vi "fetch frame gige DB1605 无点云.vi"() -> ()   [LabVIEW 2015]
uses:
  <userlib>/Mv3dRgbd/Mv3dRgbd.lvlib
  <userlib>/Mv3dRgbdEx/Mv3dRgbdEx.lvlib
panel:
  in  "设备索引":i32=5
  out "pDeviceCount out 4":u32
  out "get list return 3":i32
  out "MV3D_RGBD_GigEDEVICE_INFO out 3":T1(array[cluster])
  out "pstGigeDeviceInfo out 3":T2
  out "open gige function 2":i32
  out "start handle out":u32
  out "start function 2":i32
  in  "?":enum32{"RGBD", "点云"}(tab)
  out "二维图片":picture
  out "Depth":i16[][](graph)
  out "fetchframe function":i32
  in  "?":bool
  out "close handle out":u32
  out "close function":i32
  out "stop handle out":u32
  out "init function":i32
  out "release function":i32
  out "stop function":i32
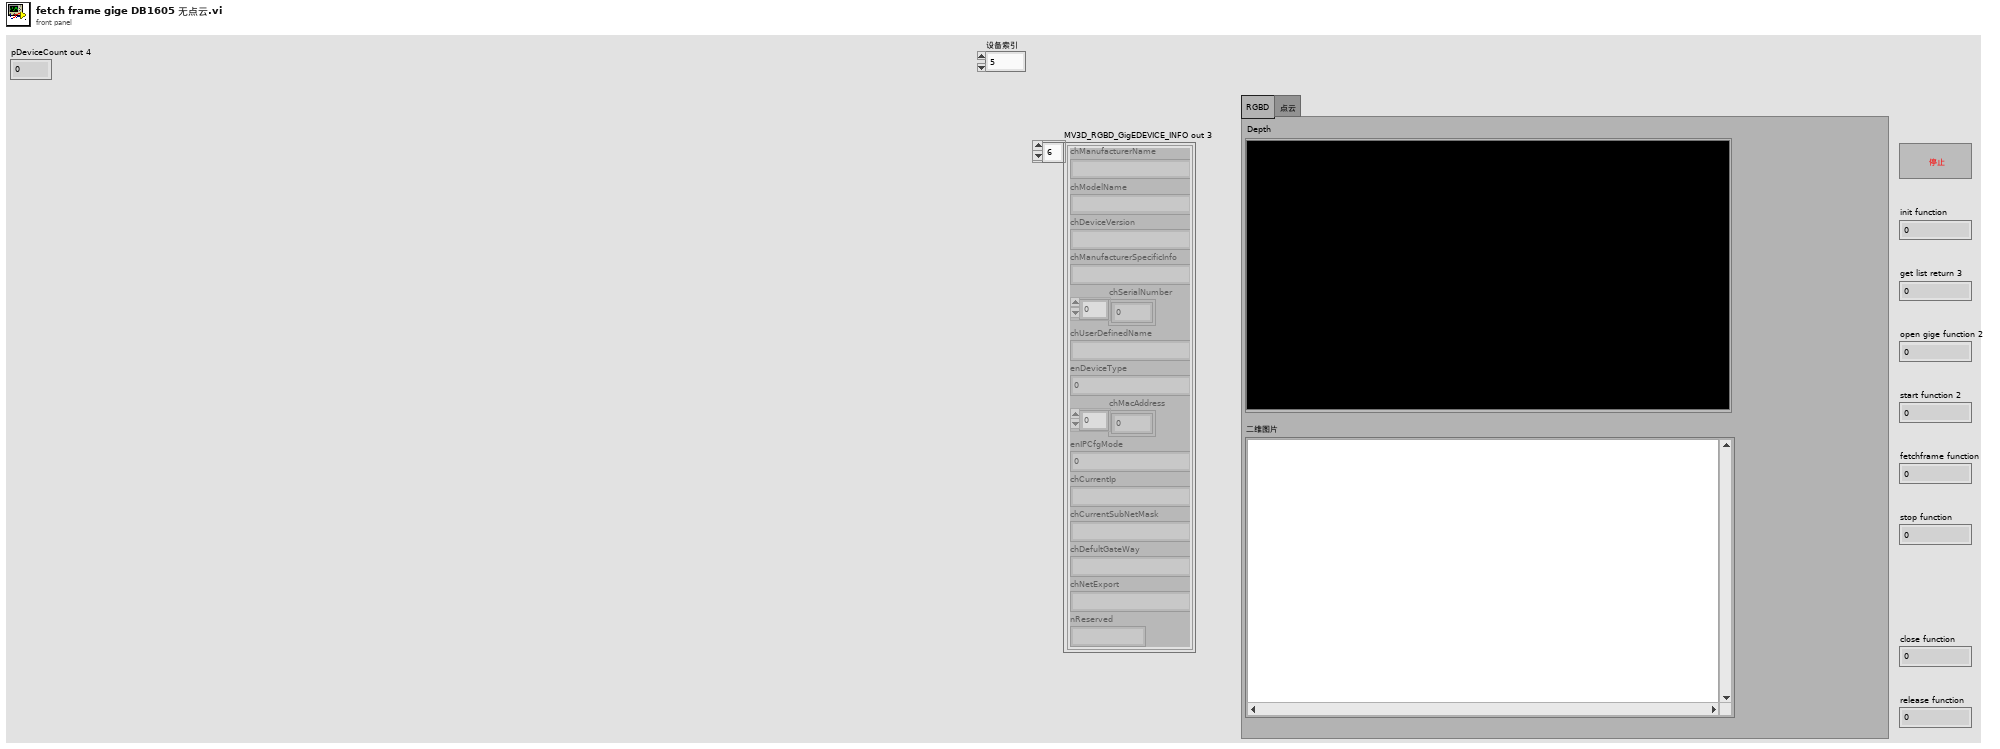
[diagram p1: front panel]
types:
  T1 = cluster{"chManufacturerName":string, "chModelName":string, "chDeviceVersion":string, "chManufacturerSpecificInfo":string, "chSerialNumber":u8[], "chUserDefinedName":string, "enDeviceType":i32, "chMacAddress":u8[], "enIPCfgMode":i32, "chCurrentIp":string, "chCurrentSubNetMask":string, "chDefultGateWay":string, "chNetExport":string, "nReserved":string}[]
  T2 = cluster{"chManufacturerName[0]":i8, "chManufacturerName[1]":i8, "chManufacturerName[2]":i8, "chManufacturerName[3]":i8, "chManufacturerName[4]":i8, "chManufacturerName[5]":i8, "chManufacturerName[6]":i8, "chManufacturerName[7]":i8, "chManufacturerName[8]":i8, "chManufacturerName[9]":i8, "chManufacturerName[10]":i8, "chManufacturerName[11]":i8, "chManufacturerName[12]":i8, "chManufacturerName[13]":i8, "chManufacturerName[14]":i8, "chManufacturerName[15]":i8, "chManufacturerName[16]":i8, "chManufacturerName[17]":i8, "chManufacturerName[18]":i8, "chManufacturerName[19]":i8, "chManufacturerName[20]":i8, "chManufacturerName[21]":i8, "chManufacturerName[22]":i8, "chManufacturerName[23]":i8, "chManufacturerName[24]":i8, "chManufacturerName[25]":i8, "chManufacturerName[26]":i8, "chManufacturerName[27]":i8, "chManufacturerName[28]":i8, "chManufacturerName[29]":i8, "chManufacturerName[30]":i8, "chManufacturerName[31]":i8, "chModelName[0]":i8, "chModelName[1]":i8, "chModelName[2]":i8, "chModelName[3]":i8, "chModelName[4]":i8, "chModelName[5]":i8, "chModelName[6]":i8, "chModelName[7]":i8, "chModelName[8]":i8, "chModelName[9]":i8, "chModelName[10]":i8, "chModelName[11]":i8, "chModelName[12]":i8, "chModelName[13]":i8, "chModelName[14]":i8, "chModelName[15]":i8, "chModelName[16]":i8, "chModelName[17]":i8, "chModelName[18]":i8, "chModelName[19]":i8, "chModelName[20]":i8, "chModelName[21]":i8, "chModelName[22]":i8, "chModelName[23]":i8, "chModelName[24]":i8, "chModelName[25]":i8, "chModelName[26]":i8, "chModelName[27]":i8, "chModelName[28]":i8, "chModelName[29]":i8, "chModelName[30]":i8, "chModelName[31]":i8, "chDeviceVersion[0]":i8, "chDeviceVersion[1]":i8, "chDeviceVersion[2]":i8, "chDeviceVersion[3]":i8, "chDeviceVersion[4]":i8, "chDeviceVersion[5]":i8, "chDeviceVersion[6]":i8, "chDeviceVersion[7]":i8, "chDeviceVersion[8]":i8, "chDeviceVersion[9]":i8, "chDeviceVersion[10]":i8, "chDeviceVersion[11]":i8, "chDeviceVersion[12]":i8, "chDeviceVersion[13]":i8, "chDeviceVersion[14]":i8, "chDeviceVersion[15]":i8, "chDeviceVersion[16]":i8, "chDeviceVersion[17]":i8, "chDeviceVersion[18]":i8, "chDeviceVersion[19]":i8, "chDeviceVersion[20]":i8, "chDeviceVersion[21]":i8, "chDeviceVersion[22]":i8, "chDeviceVersion[23]":i8, "chDeviceVersion[24]":i8, "chDeviceVersion[25]":i8, "chDeviceVersion[26]":i8, "chDeviceVersion[27]":i8, "chDeviceVersion[28]":i8, "chDeviceVersion[29]":i8, "chDeviceVersion[30]":i8, "chDeviceVersion[31]":i8, "chManufacturerSpecificInfo[0]":i8, "chManufacturerSpecificInfo[1]":i8, "chManufacturerSpecificInfo[2]":i8, "chManufacturerSpecificInfo[3]":i8, "chManufacturerSpecificInfo[4]":i8, "chManufacturerSpecificInfo[5]":i8, "chManufacturerSpecificInfo[6]":i8, "chManufacturerSpecificInfo[7]":i8, "chManufacturerSpecificInfo[8]":i8, "chManufacturerSpecificInfo[9]":i8, "chManufacturerSpecificInfo[10]":i8, "chManufacturerSpecificInfo[11]":i8, "chManufacturerSpecificInfo[12]":i8, "chManufacturerSpecificInfo[13]":i8, "chManufacturerSpecificInfo[14]":i8, "chManufacturerSpecificInfo[15]":i8, "chManufacturerSpecificInfo[16]":i8, "chManufacturerSpecificInfo[17]":i8, "chManufacturerSpecificInfo[18]":i8, "chManufacturerSpecificInfo[19]":i8, "chManufacturerSpecificInfo[20]":i8, "chManufacturerSpecificInfo[21]":i8, "chManufacturerSpecificInfo[22]":i8, "chManufacturerSpecificInfo[23]":i8, "chManufacturerSpecificInfo[24]":i8, "chManufacturerSpecificInfo[25]":i8, "chManufacturerSpecificInfo[26]":i8, "chManufacturerSpecificInfo[27]":i8, "chManufacturerSpecificInfo[28]":i8, "chManufacturerSpecificInfo[29]":i8, "chManufacturerSpecificInfo[30]":i8, "chManufacturerSpecificInfo[31]":i8, "chManufacturerSpecificInfo[32]":i8, "chManufacturerSpecificInfo[33]":i8, "chManufacturerSpecificInfo[34]":i8, "chManufacturerSpecificInfo[35]":i8, "chManufacturerSpecificInfo[36]":i8, "chManufacturerSpecificInfo[37]":i8, "chManufacturerSpecificInfo[38]":i8, "chManufacturerSpecificInfo[39]":i8, "chManufacturerSpecificInfo[40]":i8, "chManufacturerSpecificInfo[41]":i8, "chManufacturerSpecificInfo[42]":i8, "chManufacturerSpecificInfo[43]":i8, "chManufacturerSpecificInfo[44]":i8, "chManufacturerSpecificInfo[45]":i8, "chManufacturerSpecificInfo[46]":i8, "chManufacturerSpecificInfo[47]":i8, "chSerialNumber[0]":i8, "chSerialNumber[1]":i8, "chSerialNumber[2]":i8, "chSerialNumber[3]":i8, "chSerialNumber[4]":i8, "chSerialNumber[5]":i8, "chSerialNumber[6]":i8, "chSerialNumber[7]":i8, "chSerialNumber[8]":i8, "chSerialNumber[9]":i8, "chSerialNumber[10]":i8, "chSerialNumber[11]":i8, "chSerialNumber[12]":i8, "chSerialNumber[13]":i8, "chSerialNumber[14]":i8, "chSerialNumber[15]":i8, "chUserDefinedName[0]":i8, "chUserDefinedName[1]":i8, "chUserDefinedName[2]":i8, "chUserDefinedName[3]":i8, "chUserDefinedName[4]":i8, "chUserDefinedName[5]":i8, "chUserDefinedName[6]":i8, "chUserDefinedName[7]":i8, "chUserDefinedName[8]":i8, "chUserDefinedName[9]":i8, "chUserDefinedName[10]":i8, "chUserDefinedName[11]":i8, "chUserDefinedName[12]":i8, "chUserDefinedName[13]":i8, "chUserDefinedName[14]":i8, "chUserDefinedName[15]":i8, "enDeviceType":i32, "chMacAddress[0]":u8, "chMacAddress[1]":u8, "chMacAddress[2]":u8, "chMacAddress[3]":u8, "chMacAddress[4]":u8, "chMacAddress[5]":u8, "chMacAddress[6]":u8, "chMacAddress[7]":u8, "enIPCfgMode":i32, "chCurrentIp[0]":i8, "chCurrentIp[1]":i8, "chCurrentIp[2]":i8, "chCurrentIp[3]":i8, "chCurrentIp[4]":i8, "chCurrentIp[5]":i8, "chCurrentIp[6]":i8, "chCurrentIp[7]":i8, "chCurrentIp[8]":i8, "chCurrentIp[9]":i8, "chCurrentIp[10]":i8, "chCurrentIp[11]":i8, "chCurrentIp[12]":i8, "chCurrentIp[13]":i8, "chCurrentIp[14]":i8, "chCurrentIp[15]":i8, "chCurrentSubNetMask[0]":i8, "chCurrentSubNetMask[1]":i8, "chCurrentSubNetMask[2]":i8, "chCurrentSubNetMask[3]":i8, "chCurrentSubNetMask[4]":i8, "chCurrentSubNetMask[5]":i8, "chCurrentSubNetMask[6]":i8, "chCurrentSubNetMask[7]":i8, "chCurrentSubNetMask[8]":i8, "chCurrentSubNetMask[9]":i8, "chCurrentSubNetMask[10]":i8, "chCurrentSubNetMask[11]":i8, "chCurrentSubNetMask[12]":i8, "chCurrentSubNetMask[13]":i8, "chCurrentSubNetMask[14]":i8, "chCurrentSubNetMask[15]":i8, "chDefultGateWay[0]":i8, "chDefultGateWay[1]":i8, "chDefultGateWay[2]":i8, "chDefultGateWay[3]":i8, "chDefultGateWay[4]":i8, "chDefultGateWay[5]":i8, "chDefultGateWay[6]":i8, "chDefultGateWay[7]":i8, "chDefultGateWay[8]":i8, "chDefultGateWay[9]":i8, "chDefultGateWay[10]":i8, "chDefultGateWay[11]":i8, "chDefultGateWay[12]":i8, "chDefultGateWay[13]":i8, "chDefultGateWay[14]":i8, "chDefultGateWay[15]":i8, "chNetExport[0]":i8, "chNetExport[1]":i8, "chNetExport[2]":i8, "chNetExport[3]":i8, "chNetExport[4]":i8, "chNetExport[5]":i8, "chNetExport[6]":i8, "chNetExport[7]":i8, "chNetExport[8]":i8, "chNetExport[9]":i8, "chNetExport[10]":i8, "chNetExport[11]":i8, "chNetExport[12]":i8, "chNetExport[13]":i8, "chNetExport[14]":i8, "chNetExport[15]":i8, "nReserved[0]":u8, "nReserved[1]":u8, "nReserved[2]":u8, "nReserved[3]":u8, "nReserved[4]":u8, "nReserved[5]":u8, "nReserved[6]":u8, "nReserved[7]":u8, "nReserved[8]":u8, "nReserved[9]":u8, "nReserved[10]":u8, "nReserved[11]":u8, "nReserved[12]":u8, "nReserved[13]":u8, "nReserved[14]":u8, "nReserved[15]":u8}
  T3 = cluster{"chManufacturerName[0]":i8, "chManufacturerName[1]":i8, "chManufacturerName[2]":i8, "chManufacturerName[3]":i8, "chManufacturerName[4]":i8, "chManufacturerName[5]":i8, "chManufacturerName[6]":i8, "chManufacturerName[7]":i8, "chManufacturerName[8]":i8, "chManufacturerName[9]":i8, "chManufacturerName[10]":i8, "chManufacturerName[11]":i8, "chManufacturerName[12]":i8, "chManufacturerName[13]":i8, "chManufacturerName[14]":i8, "chManufacturerName[15]":i8, "chManufacturerName[16]":i8, "chManufacturerName[17]":i8, "chManufacturerName[18]":i8, "chManufacturerName[19]":i8, "chManufacturerName[20]":i8, "chManufacturerName[21]":i8, "chManufacturerName[22]":i8, "chManufacturerName[23]":i8, "chManufacturerName[24]":i8, "chManufacturerName[25]":i8, "chManufacturerName[26]":i8, "chManufacturerName[27]":i8, "chManufacturerName[28]":i8, "chManufacturerName[29]":i8, "chManufacturerName[30]":i8, "chManufacturerName[31]":i8, "chModelName[0]":i8, "chModelName[1]":i8, "chModelName[2]":i8, "chModelName[3]":i8, "chModelName[4]":i8, "chModelName[5]":i8, "chModelName[6]":i8, "chModelName[7]":i8, "chModelName[8]":i8, "chModelName[9]":i8, "chModelName[10]":i8, "chModelName[11]":i8, "chModelName[12]":i8, "chModelName[13]":i8, "chModelName[14]":i8, "chModelName[15]":i8, "chModelName[16]":i8, "chModelName[17]":i8, "chModelName[18]":i8, "chModelName[19]":i8, "chModelName[20]":i8, "chModelName[21]":i8, "chModelName[22]":i8, "chModelName[23]":i8, "chModelName[24]":i8, "chModelName[25]":i8, "chModelName[26]":i8, "chModelName[27]":i8, "chModelName[28]":i8, "chModelName[29]":i8, "chModelName[30]":i8, "chModelName[31]":i8, "chDeviceVersion[0]":i8, "chDeviceVersion[1]":i8, "chDeviceVersion[2]":i8, "chDeviceVersion[3]":i8, "chDeviceVersion[4]":i8, "chDeviceVersion[5]":i8, "chDeviceVersion[6]":i8, "chDeviceVersion[7]":i8, "chDeviceVersion[8]":i8, "chDeviceVersion[9]":i8, "chDeviceVersion[10]":i8, "chDeviceVersion[11]":i8, "chDeviceVersion[12]":i8, "chDeviceVersion[13]":i8, "chDeviceVersion[14]":i8, "chDeviceVersion[15]":i8, "chDeviceVersion[16]":i8, "chDeviceVersion[17]":i8, "chDeviceVersion[18]":i8, "chDeviceVersion[19]":i8, "chDeviceVersion[20]":i8, "chDeviceVersion[21]":i8, "chDeviceVersion[22]":i8, "chDeviceVersion[23]":i8, "chDeviceVersion[24]":i8, "chDeviceVersion[25]":i8, "chDeviceVersion[26]":i8, "chDeviceVersion[27]":i8, "chDeviceVersion[28]":i8, "chDeviceVersion[29]":i8, "chDeviceVersion[30]":i8, "chDeviceVersion[31]":i8, "chManufacturerSpecificInfo[0]":i8, "chManufacturerSpecificInfo[1]":i8, "chManufacturerSpecificInfo[2]":i8, "chManufacturerSpecificInfo[3]":i8, "chManufacturerSpecificInfo[4]":i8, "chManufacturerSpecificInfo[5]":i8, "chManufacturerSpecificInfo[6]":i8, "chManufacturerSpecificInfo[7]":i8, "chManufacturerSpecificInfo[8]":i8, "chManufacturerSpecificInfo[9]":i8, "chManufacturerSpecificInfo[10]":i8, "chManufacturerSpecificInfo[11]":i8, "chManufacturerSpecificInfo[12]":i8, "chManufacturerSpecificInfo[13]":i8, "chManufacturerSpecificInfo[14]":i8, "chManufacturerSpecificInfo[15]":i8, "chManufacturerSpecificInfo[16]":i8, "chManufacturerSpecificInfo[17]":i8, "chManufacturerSpecificInfo[18]":i8, "chManufacturerSpecificInfo[19]":i8, "chManufacturerSpecificInfo[20]":i8, "chManufacturerSpecificInfo[21]":i8, "chManufacturerSpecificInfo[22]":i8, "chManufacturerSpecificInfo[23]":i8, "chManufacturerSpecificInfo[24]":i8, "chManufacturerSpecificInfo[25]":i8, "chManufacturerSpecificInfo[26]":i8, "chManufacturerSpecificInfo[27]":i8, "chManufacturerSpecificInfo[28]":i8, "chManufacturerSpecificInfo[29]":i8, "chManufacturerSpecificInfo[30]":i8, "chManufacturerSpecificInfo[31]":i8, "chManufacturerSpecificInfo[32]":i8, "chManufacturerSpecificInfo[33]":i8, "chManufacturerSpecificInfo[34]":i8, "chManufacturerSpecificInfo[35]":i8, "chManufacturerSpecificInfo[36]":i8, "chManufacturerSpecificInfo[37]":i8, "chManufacturerSpecificInfo[38]":i8, "chManufacturerSpecificInfo[39]":i8, "chManufacturerSpecificInfo[40]":i8, "chManufacturerSpecificInfo[41]":i8, "chManufacturerSpecificInfo[42]":i8, "chManufacturerSpecificInfo[43]":i8, "chManufacturerSpecificInfo[44]":i8, "chManufacturerSpecificInfo[45]":i8, "chManufacturerSpecificInfo[46]":i8, "chManufacturerSpecificInfo[47]":i8, "chSerialNumber[0]":i8, "chSerialNumber[1]":i8, "chSerialNumber[2]":i8, "chSerialNumber[3]":i8, "chSerialNumber[4]":i8, "chSerialNumber[5]":i8, "chSerialNumber[6]":i8, "chSerialNumber[7]":i8, "chSerialNumber[8]":i8, "chSerialNumber[9]":i8, "chSerialNumber[10]":i8, "chSerialNumber[11]":i8, "chSerialNumber[12]":i8, "chSerialNumber[13]":i8, "chSerialNumber[14]":i8, "chSerialNumber[15]":i8, "chUserDefinedName[0]":i8, "chUserDefinedName[1]":i8, "chUserDefinedName[2]":i8, "chUserDefinedName[3]":i8, "chUserDefinedName[4]":i8, "chUserDefinedName[5]":i8, "chUserDefinedName[6]":i8, "chUserDefinedName[7]":i8, "chUserDefinedName[8]":i8, "chUserDefinedName[9]":i8, "chUserDefinedName[10]":i8, "chUserDefinedName[11]":i8, "chUserDefinedName[12]":i8, "chUserDefinedName[13]":i8, "chUserDefinedName[14]":i8, "chUserDefinedName[15]":i8, "enDeviceType":i32, "chMacAddress[0]":u8, "chMacAddress[1]":u8, "chMacAddress[2]":u8, "chMacAddress[3]":u8, "chMacAddress[4]":u8, "chMacAddress[5]":u8, "chMacAddress[6]":u8, "chMacAddress[7]":u8, "enIPCfgMode":i32, "chCurrentIp[0]":i8, "chCurrentIp[1]":i8, "chCurrentIp[2]":i8, "chCurrentIp[3]":i8, "chCurrentIp[4]":i8, "chCurrentIp[5]":i8, "chCurrentIp[6]":i8, "chCurrentIp[7]":i8, "chCurrentIp[8]":i8, "chCurrentIp[9]":i8, "chCurrentIp[10]":i8, "chCurrentIp[11]":i8, "chCurrentIp[12]":i8, "chCurrentIp[13]":i8, "chCurrentIp[14]":i8, "chCurrentIp[15]":i8, "chCurrentSubNetMask[0]":i8, "chCurrentSubNetMask[1]":i8, "chCurrentSubNetMask[2]":i8, "chCurrentSubNetMask[3]":i8, "chCurrentSubNetMask[4]":i8, "chCurrentSubNetMask[5]":i8, "chCurrentSubNetMask[6]":i8, "chCurrentSubNetMask[7]":i8, "chCurrentSubNetMask[8]":i8, "chCurrentSubNetMask[9]":i8, "chCurrentSubNetMask[10]":i8, "chCurrentSubNetMask[11]":i8, "chCurrentSubNetMask[12]":i8, "chCurrentSubNetMask[13]":i8, "chCurrentSubNetMask[14]":i8, "chCurrentSubNetMask[15]":i8, "chDefultGateWay[0]":i8, "chDefultGateWay[1]":i8, "chDefultGateWay[2]":i8, "chDefultGateWay[3]":i8, "chDefultGateWay[4]":i8, "chDefultGateWay[5]":i8, "chDefultGateWay[6]":i8, "chDefultGateWay[7]":i8, "chDefultGateWay[8]":i8, "chDefultGateWay[9]":i8, "chDefultGateWay[10]":i8, "chDefultGateWay[11]":i8, "chDefultGateWay[12]":i8, "chDefultGateWay[13]":i8, "chDefultGateWay[14]":i8, "chDefultGateWay[15]":i8, "chNetExport[0]":i8, "chNetExport[1]":i8, "chNetExport[2]":i8, "chNetExport[3]":i8, "chNetExport[4]":i8, "chNetExport[5]":i8, "chNetExport[6]":i8, "chNetExport[7]":i8, "chNetExport[8]":i8, "chNetExport[9]":i8, "chNetExport[10]":i8, "chNetExport[11]":i8, "chNetExport[12]":i8, "chNetExport[13]":i8, "chNetExport[14]":i8, "chNetExport[15]":i8, "nReserved[0]":u8, "nReserved[1]":u8, "nReserved[2]":u8, "nReserved[3]":u8, "nReserved[4]":u8, "nReserved[5]":u8, "nReserved[6]":u8, "nReserved[7]":u8, "nReserved[8]":u8, "nReserved[9]":u8, "nReserved[10]":u8, "nReserved[11]":u8, "nReserved[12]":u8, "nReserved[13]":u8, "nReserved[14]":u8, "nReserved[15]":u8}[]
  T4 = cluster{"nImageCount":u64, "MV3D_RGBD_IMAGE_DATA[0]":cluster{"enImageType":i32, "nWidth":u32, "nHeight":u32, "pData":u32, "nDataLen":u32, "nFrameNum":u32, "nTimeStamp":i64, "nReserved[0]":u8, "nReserved[1]":u8, "nReserved[2]":u8, "nReserved[3]":u8, "nReserved[4]":u8, "nReserved[5]":u8, "nReserved[6]":u8, "nReserved[7]":u8, "nReserved[8]":u8, "nReserved[9]":u8, "nReserved[10]":u8, "nReserved[11]":u8, "nReserved[12]":u8, "nReserved[13]":u8, "nReserved[14]":u8, "nReserved[15]":u8}, "MV3D_RGBD_IMAGE_DATA[1]":cluster{"enImageType":i32, "nWidth":u32, "nHeight":u32, "pData":u32, "nDataLen":u32, "nFrameNum":u32, "nTimeStamp":i64, "nReserved[0]":u8, "nReserved[1]":u8, "nReserved[2]":u8, "nReserved[3]":u8, "nReserved[4]":u8, "nReserved[5]":u8, "nReserved[6]":u8, "nReserved[7]":u8, "nReserved[8]":u8, "nReserved[9]":u8, "nReserved[10]":u8, "nReserved[11]":u8, "nReserved[12]":u8, "nReserved[13]":u8, "nReserved[14]":u8, "nReserved[15]":u8}, "MV3D_RGBD_IMAGE_DATA[2]":cluster{"enImageType":i32, "nWidth":u32, "nHeight":u32, "pData":u32, "nDataLen":u32, "nFrameNum":u32, "nTimeStamp":i64, "nReserved[0]":u8, "nReserved[1]":u8, "nReserved[2]":u8, "nReserved[3]":u8, "nReserved[4]":u8, "nReserved[5]":u8, "nReserved[6]":u8, "nReserved[7]":u8, "nReserved[8]":u8, "nReserved[9]":u8, "nReserved[10]":u8, "nReserved[11]":u8, "nReserved[12]":u8, "nReserved[13]":u8, "nReserved[14]":u8, "nReserved[15]":u8}, "MV3D_RGBD_IMAGE_DATA[3]":cluster{"enImageType":i32, "nWidth":u32, "nHeight":u32, "pData":u32, "nDataLen":u32, "nFrameNum":u32, "nTimeStamp":i64, "nReserved[0]":u8, "nReserved[1]":u8, "nReserved[2]":u8, "nReserved[3]":u8, "nReserved[4]":u8, "nReserved[5]":u8, "nReserved[6]":u8, "nReserved[7]":u8, "nReserved[8]":u8, "nReserved[9]":u8, "nReserved[10]":u8, "nReserved[11]":u8, "nReserved[12]":u8, "nReserved[13]":u8, "nReserved[14]":u8, "nReserved[15]":u8}, "MV3D_RGBD_IMAGE_DATA[4]":cluster{"enImageType":i32, "nWidth":u32, "nHeight":u32, "pData":u32, "nDataLen":u32, "nFrameNum":u32, "nTimeStamp":i64, "nReserved[0]":u8, "nReserved[1]":u8, "nReserved[2]":u8, "nReserved[3]":u8, "nReserved[4]":u8, "nReserved[5]":u8, "nReserved[6]":u8, "nReserved[7]":u8, "nReserved[8]":u8, "nReserved[9]":u8, "nReserved[10]":u8, "nReserved[11]":u8, "nReserved[12]":u8, "nReserved[13]":u8, "nReserved[14]":u8, "nReserved[15]":u8}, "MV3D_RGBD_IMAGE_DATA[5]":cluster{"enImageType":i32, "nWidth":u32, "nHeight":u32, "pData":u32, "nDataLen":u32, "nFrameNum":u32, "nTimeStamp":i64, "nReserved[0]":u8, "nReserved[1]":u8, "nReserved[2]":u8, "nReserved[3]":u8, "nReserved[4]":u8, "nReserved[5]":u8, "nReserved[6]":u8, "nReserved[7]":u8, "nReserved[8]":u8, "nReserved[9]":u8, "nReserved[10]":u8, "nReserved[11]":u8, "nReserved[12]":u8, "nReserved[13]":u8, "nReserved[14]":u8, "nReserved[15]":u8}, "MV3D_RGBD_IMAGE_DATA[6]":cluster{"enImageType":i32, "nWidth":u32, "nHeight":u32, "pData":u32, "nDataLen":u32, "nFrameNum":u32, "nTimeStamp":i64, "nReserved[0]":u8, "nReserved[1]":u8, "nReserved[2]":u8, "nReserved[3]":u8, "nReserved[4]":u8, "nReserved[5]":u8, "nReserved[6]":u8, "nReserved[7]":u8, "nReserved[8]":u8, "nReserved[9]":u8, "nReserved[10]":u8, "nReserved[11]":u8, "nReserved[12]":u8, "nReserved[13]":u8, "nReserved[14]":u8, "nReserved[15]":u8}, "MV3D_RGBD_IMAGE_DATA[7]":cluster{"enImageType":i32, "nWidth":u32, "nHeight":u32, "pData":u32, "nDataLen":u32, "nFrameNum":u32, "nTimeStamp":i64, "nReserved[0]":u8, "nReserved[1]":u8, "nReserved[2]":u8, "nReserved[3]":u8, "nReserved[4]":u8, "nReserved[5]":u8, "nReserved[6]":u8, "nReserved[7]":u8, "nReserved[8]":u8, "nReserved[9]":u8, "nReserved[10]":u8, "nReserved[11]":u8, "nReserved[12]":u8, "nReserved[13]":u8, "nReserved[14]":u8, "nReserved[15]":u8}, "MV3D_RGBD_IMAGE_DATA[8]":cluster{"enImageType":i32, "nWidth":u32, "nHeight":u32, "pData":u32, "nDataLen":u32, "nFrameNum":u32, "nTimeStamp":i64, "nReserved[0]":u8, "nReserved[1]":u8, "nReserved[2]":u8, "nReserved[3]":u8, "nReserved[4]":u8, "nReserved[5]":u8, "nReserved[6]":u8, "nReserved[7]":u8, "nReserved[8]":u8, "nReserved[9]":u8, "nReserved[10]":u8, "nReserved[11]":u8, "nReserved[12]":u8, "nReserved[13]":u8, "nReserved[14]":u8, "nReserved[15]":u8}, "MV3D_RGBD_IMAGE_DATA[9]":cluster{"enImageType":i32, "nWidth":u32, "nHeight":u32, "pData":u32, "nDataLen":u32, "nFrameNum":u32, "nTimeStamp":i64, "nReserved[0]":u8, "nReserved[1]":u8, "nReserved[2]":u8, "nReserved[3]":u8, "nReserved[4]":u8, "nReserved[5]":u8, "nReserved[6]":u8, "nReserved[7]":u8, "nReserved[8]":u8, "nReserved[9]":u8, "nReserved[10]":u8, "nReserved[11]":u8, "nReserved[12]":u8, "nReserved[13]":u8, "nReserved[14]":u8, "nReserved[15]":u8}, "nReserved[0]":u8, "nReserved[1]":u8, "nReserved[2]":u8, "nReserved[3]":u8, "nReserved[4]":u8, "nReserved[5]":u8, "nReserved[6]":u8, "nReserved[7]":u8, "nReserved[8]":u8, "nReserved[9]":u8, "nReserved[10]":u8, "nReserved[11]":u8, "nReserved[12]":u8, "nReserved[13]":u8, "nReserved[14]":u8, "nReserved[15]":u8}
  T5 = cluster{"enImageType":i32, "nWidth":u32, "nHeight":u32, "pData":u32, "nDataLen":u32, "nFrameNum":u32, "nTimeStamp":i64, "nReserved[0]":u8, "nReserved[1]":u8, "nReserved[2]":u8, "nReserved[3]":u8, "nReserved[4]":u8, "nReserved[5]":u8, "nReserved[6]":u8, "nReserved[7]":u8, "nReserved[8]":u8, "nReserved[9]":u8, "nReserved[10]":u8, "nReserved[11]":u8, "nReserved[12]":u8, "nReserved[13]":u8, "nReserved[14]":u8, "nReserved[15]":u8}
  T6 = typedef "imagedata.ctl" = cluster{"image type":i32, "image depth":i32, "image":u8[], "mask":u8[], "colors":u32[], "Rectangle":cluster{"left":i16, "top":i16, "right":i16, "bottom":i16}}
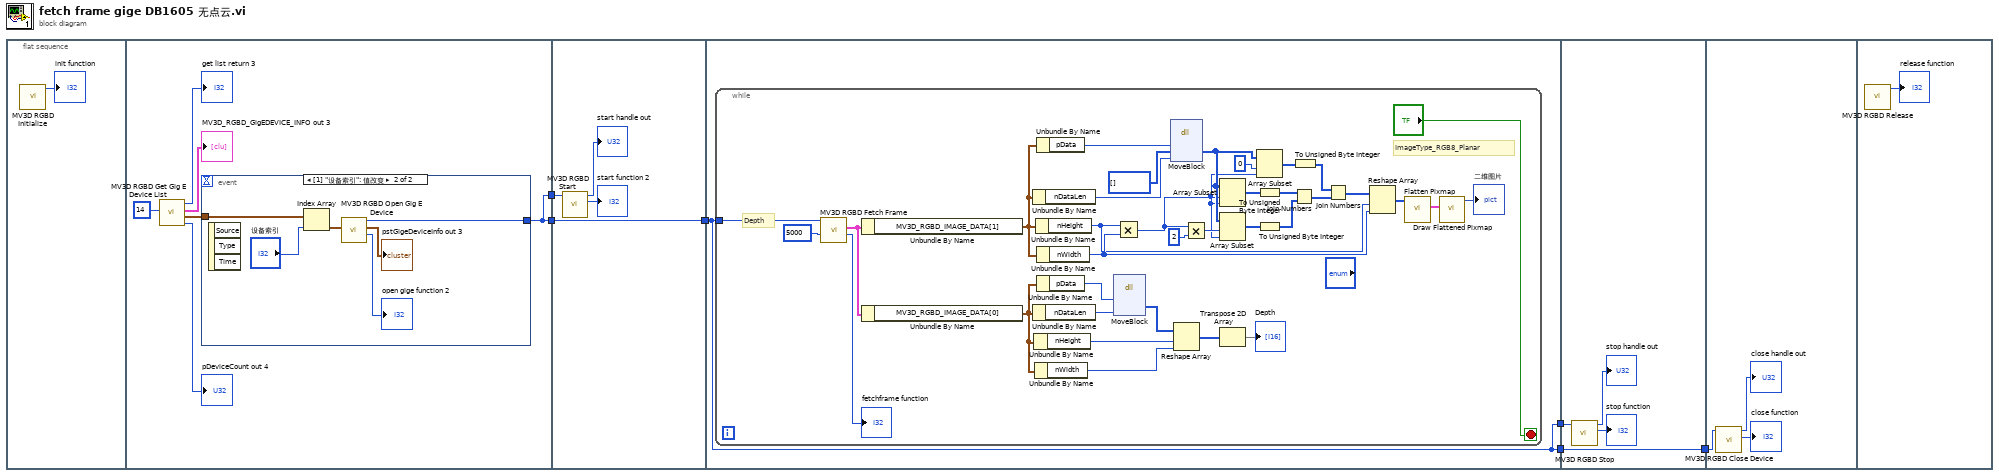
[diagram p0: block diagram]
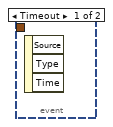
[diagram p2: hidden frame]
diagram:
  n1 = flat-sequence {
    tunnel: [w8] -> w3
    tunnel: [w8] -> w2
    tunnel: w3 -> [w21]
    tunnel: w2 -> [w20]
    tunnel: [w20] -> w1
    tunnel: [w24] -> w5
    tunnel: [w24] -> w4
    tunnel: w1 -> [w24]
    tunnel: [w60] -> w6
    tunnel: w5 -> [w60]
    tunnel: w4 -> [w61]
    tunnel: w6 -> [w64]
    frame #0 {
      n2 = call <userlib>:"MV3D RGBD Initialize.vi"() -> ("function return"=→"init function":i32)  [unwired: 11 in]
    }
    frame #1 {
      n3 = call <userlib>:"MV3D RGBD Get Gig E Device List.vi"("nMaxDeviceCount"=u32 14) -> ("pDeviceCount out"=→"pDeviceCount out 4":u32, "MV3D_RGBD_GigEDEVICE_ByteINFO out"=w9:T3, "MV3D_RGBD_GigEDEVICE_INFO out"=→"MV3D_RGBD_GigEDEVICE_INFO out 3":T1, "function return"=→"get list return 3":i32)  [unwired: 7 in]
      n4 = event shown="[1] \"设备索引\": 值改变" {
        selector: _ -> [_ _]
        dyn-events: _ -> [_ _]
        timeout: _ -> [_ _]
        tunnel: w9 -> [_ w15]
        tunnel: [_ w14] -> w8
        event Timeout {
          n5 = event-data() -> ()  [unwired: 1 in, 3 out]
        }
        event "设备索引": Value Change {
          n6 = event-data() -> ()  [unwired: 1 in, 3 out]
          n7 = Index Array(array=w15, index="设备索引") -> (element=w17:T2)
          n8 = call <userlib>:"MV3D RGBD Open Gig E Device.vi"("pstGigeDeviceInfo 2"=w17) -> ("handle out"=w14:u32, "pstGigeDeviceInfo out"=→"pstGigeDeviceInfo out 3":T2, "function return"=→"open gige function 2":i32)  [unwired: 7 in]
        }
      }
    }
    frame #2 {
      n9 = call <userlib>:"MV3D RGBD Start.vi"("handle"=w21) -> ("function return"=→"start function 2":i32, "handle out"=→"start handle out":u32)  [unwired: 9 in]
    }
    frame #3 {
      n10 = while {
        tunnel: w24 -> [w56]
        stop <- "?" stop-if-true
        # "Depth"
        # "ImageType_RGB8_Planar"
        n11 = call <userlib>:"MV3D RGBD Fetch Frame.vi"("nTimeOut"=u32 5000, "handle"=w56) -> ("function return"=→"fetchframe function":i32, "pstFrameData out"=w55:T4)  [unwired: 7 in, 1 out]
        n12 = Unbundle By Name(w55) -> ("MV3D_RGBD_IMAGE_DATA[1]"=w34:T5)
        n13 = Unbundle By Name(w55) -> ("MV3D_RGBD_IMAGE_DATA[0]"=w47:T5)
        n14 = Unbundle By Name(w34) -> ("nDataLen"=w28:u32)
        n15 = Unbundle By Name(w47) -> ("nDataLen"=w53:u32)
        n16 = Unbundle By Name(w47) -> ("nHeight"=w51:u32)
        n17 = Unbundle By Name(w47) -> ("nWidth"=w52:u32)
        n18 = Unbundle By Name(w34) -> ("nHeight"=w27:u32)
        n19 = Unbundle By Name(w34) -> ("pData"=w46:u32)
        n20 = Unbundle By Name(w34) -> ("nWidth"=w29:u32)
        n21 = Unbundle By Name(w47) -> ("pData"=w54:u32)
        n22 = dll-call lib="LabVIEW" fn="MoveBlock"("address"=w54, "size"=w53) -> ("value"=w50:i16[])  [unwired: 7 in, 2 out]
        n23 = Multiply(x=w27, y=w29) -> (x*y=w26:u32)
        n24 = dll-call lib="LabVIEW" fn="MoveBlock"("address"=w46, "value"=i16[] [] ("value 5"), "size"=w28) -> ("value"=w43:u8[])  [unwired: 6 in, 2 out]
        n25 = Reshape Array(w50, w51, w52) -> (w49:i16[][])
        n26 = Multiply(x=w26, y=u32 2) -> (x*y=w45:u32)
        n27 = Array Subset(array=w43, index=w26, length=w26) -> (w32:u8[])
        n28 = Array Subset(array=w43, index=w45, length=w26) -> (w31:u8[])
        n29 = Transpose 2D Array(2D array=w49) -> (transposed array=→"Depth":i16[][])
        n30 = Array Subset(array=w43, index=0 ("索引"), length=w26) -> (w33:u8[])
        n31 = To Unsigned Byte Integer(number=w32) -> (unsigned 8bit integer=w38:u8[])
        n32 = To Unsigned Byte Integer(number=w31) -> (unsigned 8bit integer=w35:u8[])
        n33 = Join Numbers(hi=w38, lo=w35) -> ((hi.lo)=w37:u16[])
        n34 = To Unsigned Byte Integer(number=w33) -> (unsigned 8bit integer=w36:u8[])
        n35 = Join Numbers(hi=w36, lo=w37) -> ((hi.lo)=w40:u32[])
        n36 = Reshape Array(w40, w27, w29) -> (w39:u32[][])
        n37 = call <vilib>:"Flatten Pixmap.vi"("24-bit pixmap"=w39) -> ("image data"=w25:T6)  [unwired: 10 in]
        n38 = call <vilib>:"Draw Flattened Pixmap.vi"("image data"=w25) -> ("new picture"=→"二维图片":picture)  [unwired: 8 in]
      }
    }
    frame #4 {
      n39 = call <userlib>:"MV3D RGBD Stop.vi"("handle"=w61) -> ("function return"=→"stop function":i32, "handle out"=→"stop handle out":u32)  [unwired: 9 in]
    }
    frame #5 {
      n40 = call <userlib>:"MV3D RGBD Close Device.vi"("handle"=w64) -> ("function return"=→"close function":i32, "handle out"=→"close handle out":u32)  [unwired: 9 in]
    }
    frame #6 {
      n41 = call <userlib>:"MV3D RGBD Release.vi"() -> ("function return"=→"release function":i32)  [unwired: 11 in]
    }
  }
